vi "RF Rec Configure Signal.vi"   [LabVIEW 2018]
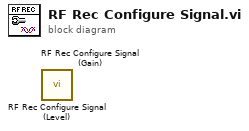
[diagram p0: block diagram]
diagram:
  n1 = call "RF Rec Configure Signal (Level).vi"() -> ()  [unwired: 9 in, 7 out]
  n2 = call "RF Rec Configure Signal (Gain).vi"() -> ()  [unwired: 9 in, 7 out]
